vi "Reset XY Graph.vi"(8 "error in (no error)":errorcluster, 11 "XYGraph in":refnum<vi>) -> (0 "error out":errorcluster)   [LabVIEW 2016]
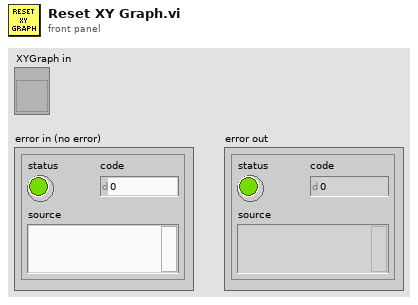
[diagram p1: front panel]
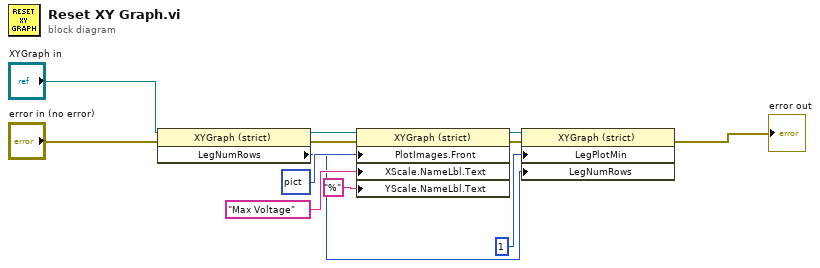
[diagram p0: block diagram]
diagram:
  n1 = property class="XYGraph (strict)"(reference="XYGraph in", error in="error in (no error)") -> (reference out=w8:refnum<vi>, error out=w6:errorcluster, "LegNumRows"=w3:u32)
  n2 = property on="Property Node" class="XYGraph (strict)"(reference=w8, error in=w6, "PlotImages.Front"=picture data[5B] ("Plot Images:Front"), "XScale.NameLbl.Text"="Max Voltage" ("X Scale.Name Label.Text"), "YScale.NameLbl.Text"="%" ("Y Scale.Name Label.Text")) -> (reference out=w2:refnum<vi>, error out=w1:errorcluster)
  n3 = property on="Property Node" class="XYGraph (strict)"(reference=w2, error in=w1, "LegPlotMin"=u32 1 ("Legend:Plot Minimum"), "LegNumRows"=w3) -> (error out=→"error out":errorcluster)  [unwired: 1 out]
